vi "4134 Read Controllers.vi"(8 "Remote 2 Packet":string, 9 "Remote 1 Packet":string, 11 "NXT":T3) -> (0 "Controller 2 State":T1={"Left X"=0, "Left Y"=0, "Right X"=0, "Right Y"=0, "Button Encoding 9-12"=0, "Button Encoding 1-8"=0, "POV"=-1} {"POV" items=["None"=-1, "POV Up"=0, "POV Up Right"=1, "POV Right"=2, "POV Down Right"=3, "POV Down"=4, "POV Down Left"=5, "POV Left"=6, "POV Up Left"=7]}, 1 "Controller 1 State":T1={"Left X"=0, "Left Y"=0, "Right X"=0, "Right Y"=0, "Button Encoding 9-12"=0, "Button Encoding 1-8"=0, "POV"=-1} {"POV" items=["None"=-1, "POV Up"=0, "POV Up Right"=1, "POV Right"=2, "POV Down Right"=3, "POV Down"=4, "POV Down Left"=5, "POV Left"=6, "POV Up Left"=7]}, 3 "NXT":T3)   [LabVIEW 2012, in "FTC.lvlib" / "Remote Interface.lvlib"]
uses:
  Remote Interface.lvlib
  <vilib>/NXT/Subs/LVHSConnector.ctl
  <vilib>/NXT/LegoClasses/BrickReference/BrickReference.lvclass
  <vilib>/FTC/FTC ControllerState.ctl
  <vilib>/FTC/FTC POVState.ctl
  Autonomous/Packet Recorder.lvlib
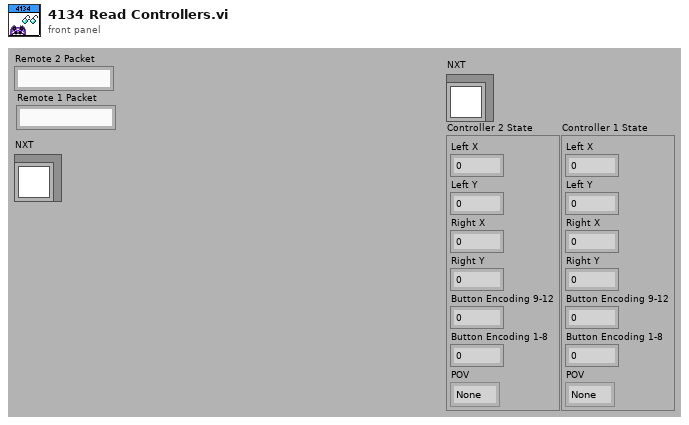
[diagram p1: front panel]
types:
  T1 = typedef "FTC ControllerState.ctl" = cluster{"Left X":i8, "Left Y":i8, "Right X":i8, "Right Y":i8, "Button Encoding 9-12":u8, "Button Encoding 1-8":u8, "POV":T2}
  T2 = typedef "FTC POVState.ctl" = i8
  T3 = typedef "LVHSConnector.ctl" = refnum<class "BrickReference.lvclass">
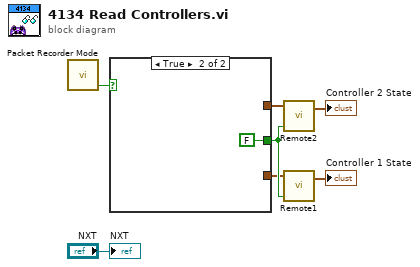
[diagram p0: block diagram]
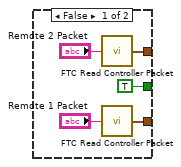
[diagram p2: hidden frame]
diagram:
  n1 = call "Packet Recorder Mode.vi"() -> ("Reading?"=w1:bool)  [unwired: 4 in, 1 out]
  n2 = case shown="True" w1 {
    tunnel: [TRUE ("Write?") FALSE ("Write?")] -> w6
    tunnel: [w10 _] -> w5
    tunnel: [w8 _] -> w4
    frame False {
      n3 = call <vilib>:"FTC Read Controller Packet.vi"("Packet"="Remote 2 Packet") -> ("Controller State"=w8:T1)  [unwired: 4 in]
      n4 = call <vilib>:"FTC Read Controller Packet.vi"("Packet"="Remote 1 Packet") -> ("Controller State"=w10:T1)  [unwired: 4 in]
    }
    frame True {
    }
  }
  n5 = call "Remote2.vi"("Write?"=w6, "Write Controller State"=w4) -> ("Controller State"=→"Controller 2 State":T1)  [unwired: 2 in]
  n6 = call "Remote1.vi"("Write?"=w6, "Write Controller State"=w5) -> ("Controller State"=→"Controller 1 State":T1)  [unwired: 2 in]
  "NXT" <- "NXT"
